vi "LVIS_Restore.vi"(8 "Error In":errorcluster, 11 "Online? In":bool) -> (0 "Error Out":errorcluster, 3 "Online? Out":bool)   [LabVIEW 2015]
doc: "Sends all data in the backup file to the Data Commander."
uses:
  Ctrls/LVIS_Msg State.ctl
  Globals/LVIS_IsGlobal.vi
  Globals/LVIS_DcGlobals.vi
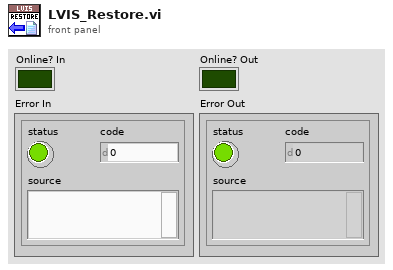
[diagram p1: front panel]
types:
  T1 = typedef "LVIS_Msg State.ctl" = enum16{"None", "Offline", "Online", "Backup Full"}
  T2 = cluster{"DCIP":string, "BackupFile":string, "ErrorLog":string, "FilePosition":string}
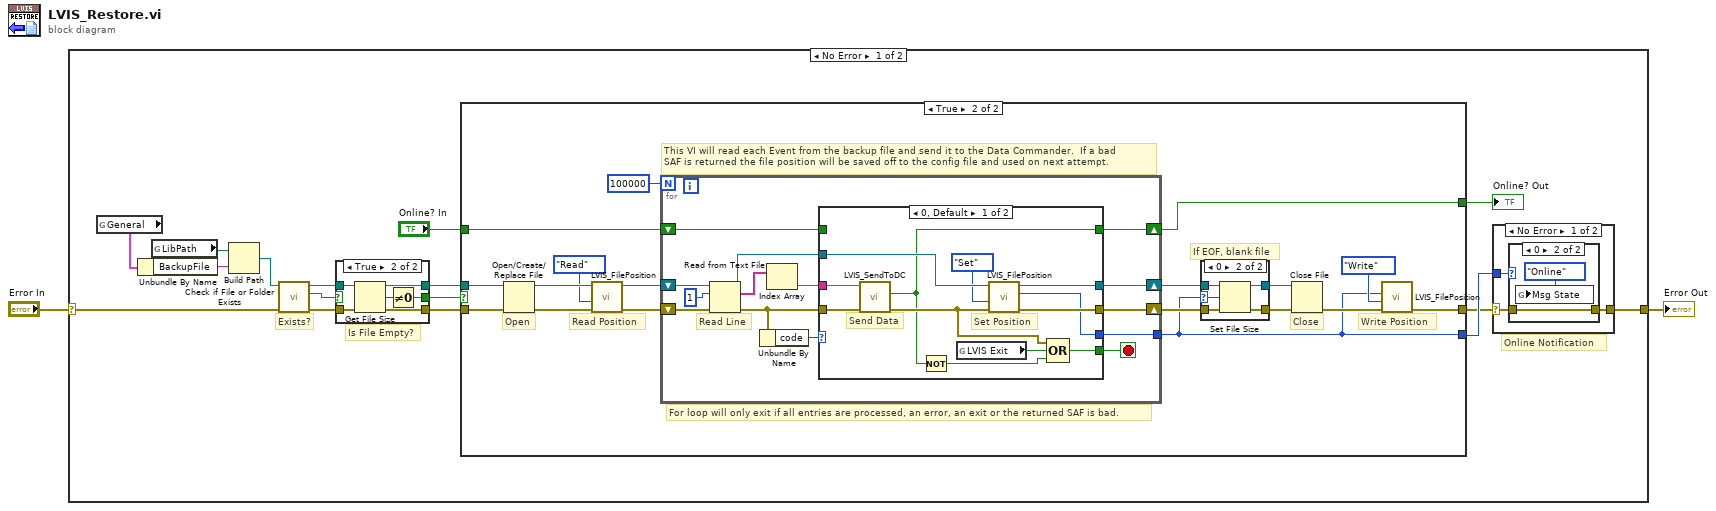
[diagram p0: block diagram]
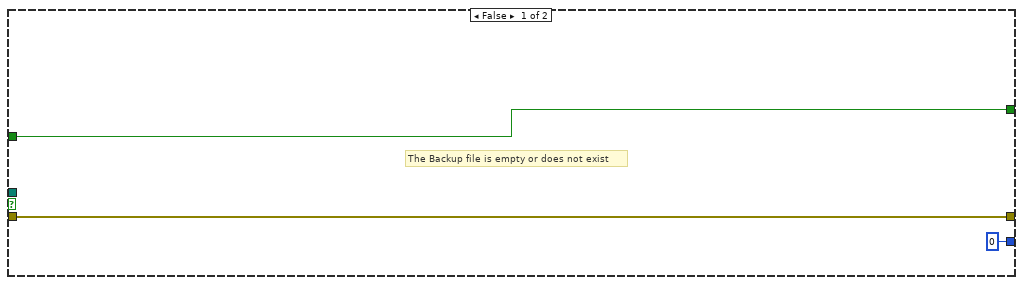
[diagram p5: hidden frame]
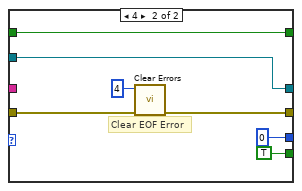
[diagram p7: hidden frame]
diagram:
  n1 = case shown="No Error" "Error In" {
    selector: "Error In" -> [w17 w95]
    tunnel: [w18 w95] -> w1
    frame No Error {
      # "Is File Empty?"
      # "Online Notification"
      # "Exists?"
      n2 = global read "LVIS_DcGlobals.vi" "General"() -> (w8:T2)
      n3 = Unbundle By Name(w8) -> ("BackupFile"=w9:string)
      n4 = global read "LVIS_IsGlobal.vi" "LibPath"() -> (w7:path)
      n5 = Build Path(base path=w7, name or relative path=w9) -> (appended path=w6:path)
      n6 = call <vilib>:"Check if File or Folder Exists.vi"("error in (no error)"=w17, "path"=w6) -> ("error out"=w12:errorcluster, "file or folder exists?"=w5:bool, "dup path"=w10:path)  [unwired: 7 in]
      n7 = case shown="True" w5 {
        selector: w5 -> [w19 _]
        tunnel: w12 -> [w20 w26]
        tunnel: [w20 w25] -> w11
        tunnel: w10 -> [w21 w22]
        tunnel: [w19 w23] -> w4
        tunnel: [w21 w22] -> w3
        frame False {
        }
        frame True {
          n8 = Get File Size(file=w22, error in=w26) -> (size (in bytes)=w24:i64, 0:w25:errorcluster)  [unwired: 1 out]
          n9 = Not Equal To 0?(x=w24) -> (x != 0?=w23:bool)
        }
      }
      n10 = case shown="True" w4 {
        tunnel: w11 -> [w36 w53]
        tunnel: [w36 w45] -> w15
        tunnel: [0 ("offset (in bytes)") w40] -> w16
        tunnel: "Online? In" -> [w34 w38]
        tunnel: [w34 w39] -> w13
        tunnel: w3 -> [_ w37]
        frame False {
          # "The Backup file is empty or does not exist"
        }
        frame True {
          # "For loop will only exit if all entries are processed, an error, an exit or the returned SAF is bad."
          # "This VI will read each Event from the backup file and send it to the Data Commander.  If a bad\nSAF is returned the file position will be saved off to the config file and used on next attempt."
          # "If EOF, blank file"
          # "Write Position"
          # "Close"
          # "Read Position"
          # "Open"
          n11 = Open/Create/Replace File(file path (use dialog)=w37, error in=w53) -> (refnum out=w50:refnum<file>, error out=w52:errorcluster)  [unwired: 4 in, 1 out]
          n12 = call "LVIS_FilePosition.vi"("Error In"=w52, "Action"=enum16{"Read", "Write", "Set"}."Read", "Ref In"=w50) -> ("Error out"=w51:errorcluster, "Ref Out"=w49:refnum<file>)  [unwired: 6 in, 1 out]
          n13 = for {
            N: 100000 -> [_]
            shift-right: [w73] -> w44
            shift-left: w51 -> [w71]
            shift-right: [w72] -> w42
            shift-left: w49 -> [w70]
            tunnel: [w66] -> w40
            shift-right: [w63] -> w39
            shift-left: w38 -> [w62]
            stop <- w69 stop-if-true
            # "Read Line"
            n14 = Read from Text File(file (use dialog)=w70, count=1, error in=w71) -> (refnum out=w74:refnum<file>, text=w68:string[], error out=w64:errorcluster)  [unwired: 1 in, 1 out]
            n15 = Unbundle By Name(w64) -> ("code"=w65:i32)
            n16 = Index Array(array=w68) -> (element=w67:string)  [unwired: 1 in]
            n17 = case shown="0, Default" w65 {
              tunnel: w74 -> [w84 w94]
              tunnel: [w85 w88] -> w73
              tunnel: [w83 w94] -> w72
              tunnel: [w86 TRUE] -> w69
              tunnel: w67 -> [w87 _]
              tunnel: [w82 0 ("offset (in bytes)")] -> w66
              tunnel: w64 -> [w80 w90]
              tunnel: [w76 w89] -> w63
              tunnel: w62 -> [_ w89]
              frame 0, Default {
                # "Set Position"
                # "Send Data"
                n18 = call "LVIS_SendToDC.vi"("Error In"=w80, "Data"=w87) -> ("Error out"=w78:errorcluster, "Online?"=w76:bool)  [unwired: 7 in, 1 out]
                n19 = Not(x=w76) -> (.not. x?=w77:bool)
                n20 = global read "LVIS_DcGlobals.vi" "LVIS Exit"() -> (w79:bool)
                n21 = call "LVIS_FilePosition.vi"("Error In"=w78, "Action"=enum16{"Read", "Write", "Set"}."Set", "Ref In"=w84) -> ("Error out"=w85:errorcluster, "Position Out"=w82:i32, "Ref Out"=w83:refnum<file>)  [unwired: 6 in]
                n22 = Compound Arithmetic op=OR(w78, w79, w77) -> (w86:bool)
              }
              frame 4 {
                # "Clear EOF Error"
                n23 = call <vilib>:"Clear Errors.vi"("error in (no error)"=w90, "specific error code to clear (0: all)"=4) -> ("error out"=w88:errorcluster)  [unwired: 4 in, 1 out]
              }
            }
          }
          n24 = case shown="0" w40 {
            selector: w40 -> [_ w57]
            tunnel: w44 -> [w56 w61]
            tunnel: [w56 w60] -> w43
            tunnel: w42 -> [w55 w59]
            tunnel: [w55 w58] -> w41
            frame 1, Default {
            }
            frame 0 {
              n25 = Set File Size(4:w61, 6:w57, 7:w59) -> (0:w60:errorcluster, 3:w58:refnum<file>)
            }
          }
          n26 = Close File(refnum=w41, error in=w43) -> (error out=w47:errorcluster)  [unwired: 1 out]
          n27 = call "LVIS_FilePosition.vi"("Error In"=w47, "Action"=enum16{"Read", "Write", "Set"}."Write", "Position In"=w40) -> ("Error out"=w45:errorcluster)  [unwired: 6 in, 2 out]
        }
      }
      "Online? Out" <- w13
      n28 = case shown="No Error" w15 {
        selector: w15 -> [w27 w33]
        tunnel: [w29 w33] -> w18
        tunnel: w16 -> [w28 _]
        frame No Error {
          n29 = case shown="0" w28 {
            tunnel: [w30 w32] -> w29
            tunnel: w27 -> [w30 w32]
            frame 1, Default {
            }
            frame 0 {
              n30 = global write "LVIS_DcGlobals.vi" "Msg State"(LVIS_Msg_State."Online" ("Msg State")) -> ()
            }
          }
        }
        frame Error {
        }
      }
    }
    frame Error {
    }
  }
  "Error Out" <- w1
